vi "NI VeriStand - FPGA PWM Out f+DC.vi"(9 "Duty Cycle":u32, 11 "Frequency":u32) -> (3 "Output":bool)   [LabVIEW 2014]
doc: "This VI generates a PWM output with Frequency and Duty Cycle."
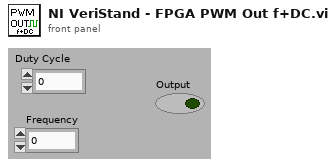
[diagram p1: front panel]
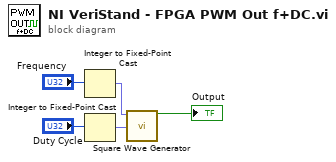
[diagram p0: block diagram]
diagram:
  n1 = Integer to Fixed-Point Cast(integer="Frequency") -> (fixed-point=w5:fxp<+,32,0>)  [unwired: 1 in]
  n2 = Integer to Fixed-Point Cast(integer="Duty Cycle") -> (fixed-point=w3:fxp<+,32,0>)  [unwired: 1 in]
  n3 = call "Square Wave Generator"("frequency (periods/tick)"=w5, "duty cycle (periods)"=w3) -> ("square wave out"=→"Output":bool)  [unwired: 13 in]
